vi "IVI-Content.vi"() -> (0 "CS++Classes & Messages":T1(array[cluster]))   [LabVIEW 2015]
doc: "Place actor and class constants that should be included included in an application on the blockdiagramm."
uses:
  <vilib>/ActorFramework/Message/Message.lvclass
  IVI_ACPwr/IVI_ACPwr.lvclass
  IVI_Counter/IVI_Counter.lvclass
  IVI_DCPwr/IVI_DCPwr.lvclass
  IVI_DMM/IVI_DMM.lvclass
  IVI_Fgen/IVI_Fgen.lvclass
  IVI_PwrMeter/IVI_PwrMeter.lvclass
  IVI_Scope/IVI_Scope.lvclass
  IVI_DMM-3458A/IVI_DMM-3458A.lvclass
  CSPP_Core/Actors/CS++BaseActor/CS++BaseActor.lvclass
panel:
  # "Place actor and class constants on the blockdiagramm."
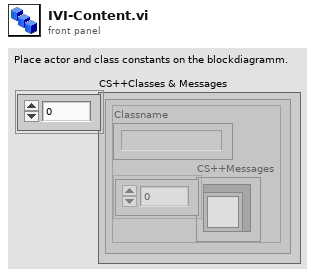
[diagram p1: front panel]
types:
  T1 = cluster{"Classname":string, "CS++Messages":refnum<class "Message.lvclass">[]}[]
  T2 = cluster{"class name":string, "CS++Messages":refnum<class "Message.lvclass">[]}
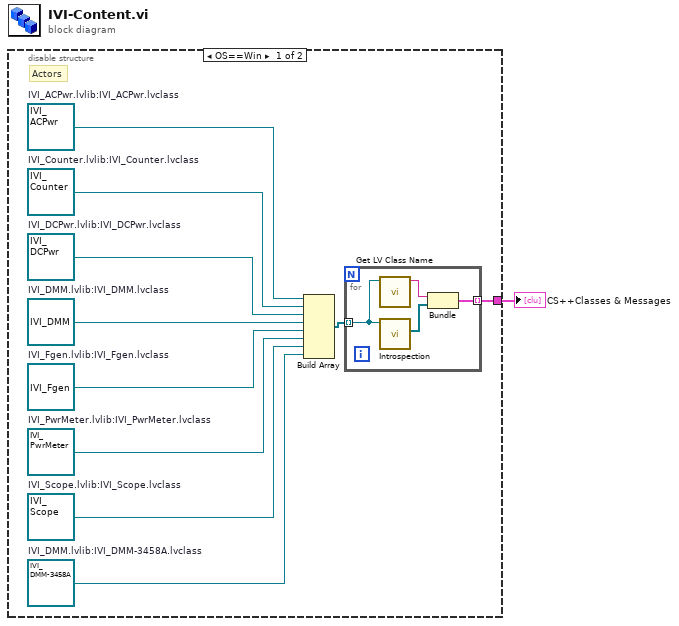
[diagram p0: block diagram]
diagram:
  n1 = disable-structure shown="OS==Win" {
    disable-tunnel: [w4 _] -> w1
    frame condition #0 (active) {
      w2 = refnum<class "IVI_DMM-3458A.lvclass"> refnum  # IVI_DMM.lvlib:IVI_DMM-3458A.lvclass
      w5 = refnum<class "IVI_Scope.lvclass"> refnum  # IVI_Scope.lvlib:IVI_Scope.lvclass
      w6 = refnum<class "IVI_PwrMeter.lvclass"> refnum  # IVI_PwrMeter.lvlib:IVI_PwrMeter.lvclass
      w7 = refnum<class "IVI_Fgen.lvclass"> refnum  # IVI_Fgen.lvlib:IVI_Fgen.lvclass
      w8 = refnum<class "IVI_DMM.lvclass"> refnum  # IVI_DMM.lvlib:IVI_DMM.lvclass
      w9 = refnum<class "IVI_DCPwr.lvclass"> refnum  # IVI_DCPwr.lvlib:IVI_DCPwr.lvclass
      w10 = refnum<class "IVI_Counter.lvclass"> refnum  # IVI_Counter.lvlib:IVI_Counter.lvclass
      w11 = refnum<class "IVI_ACPwr.lvclass"> refnum  # IVI_ACPwr.lvlib:IVI_ACPwr.lvclass
      # "Actors"
      n2 = Build Array(w11, w10, w9, w8, w7, w6, w5, w2) -> (w3:refnum<class "CS++DeviceActor.lvclass">[])
      n3 = for {
        tunnel: w3 -> [w15] mode=indexing
        tunnel: [w12] -> w4 mode=indexing
        n4 = call <vilib>:"Get LV Class Name.vi"("object"=w15) -> ("class name"=w14:string)  [unwired: 9 in, 1 out]
        n5 = call "Introspection.vi"("CS++BaseActor in"=w15) -> ("CS++Messages"=w13:refnum<class "Message.lvclass">[])  [unwired: 8 in, 2 out]
        n6 = Bundle("class name"=w14, "CS++Messages"=w13) -> (w12:T2)  [unwired: 1 in]
      }
    }
    frame condition #1 {
    }
  }
  "CS++Classes & Messages" <- w1
